vi "Disabled.vi"(7 "Robot Mode":T2, 10 "Match Info":T1={"Autonomous Elapsed Seconds"=0.0, "TeleOp Elapsed Seconds"=0.0, "Disabled Elapsed Seconds"=0.0, "Visited Autonomous"=FALSE, "Visited TeleOp"=FALSE, "Visited Disabled"=FALSE, "Autonomous Settings"={"Autonomous Style"=enum."Independent", "VI Refnum"=refnum}}, 11 "Call Context":T3) -> ()   [LabVIEW 2013]
doc: "This VI is called each time a disabled packet is received from the DS. It is often used to prepare for the next robot mode, to calibrate sensors, etc."
uses:
  <vilib>/Rock Robotics/WPI/DriverStation/WPI_DriverStationDerivedRobotMode.ctl
  <vilib>/Rock Robotics/WPI/DriverStation/WPI_DriverStationRobotMode2.ctl
  <vilib>/Rock Robotics/WPI/DriverStation/WPI_DriverStationMatch Info.ctl
  Rollers/Roller Control.ctl
  Rollers/Roller Mode.ctl
  Common Code/Change Detect Boolean.vi
  <vilib>/Rock Robotics/WPI/Joystick/WPI_JoystickRefNum Registry Get.vi
  Utilities/Invert Joystick Y Axes.vi
  Drivetrain/Drivetrain Set.vi
  Robot Global Data.vi
  <vilib>/Rock Robotics/WPI/Joystick/WPI_JoystickGet.vi
  <vilib>/Rock Robotics/WPI/Joystick/WPI_JoystickGetSetRefNum.vi
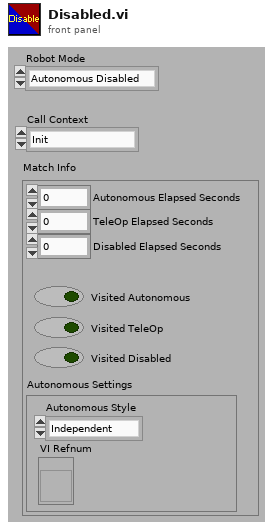
[diagram p1: front panel]
types:
  T1 = typedef "WPI_DriverStationMatch Info.ctl" = cluster{"Autonomous Elapsed Seconds":dbl, "TeleOp Elapsed Seconds":dbl, "Disabled Elapsed Seconds":dbl, "Visited Autonomous":bool, "Visited TeleOp":bool, "Visited Disabled":bool, "Autonomous Settings":cluster{"Autonomous Style":enum16{"Iterative", "Independent"}, "VI Refnum":refnum<vi>}}
  T2 = typedef "WPI_DriverStationRobotMode2.ctl" = enum16{"Autonomous Disabled", "Autonomous Enabled", "Teleop Disabled", "Teleop Enabled", "Timeout", "Finish", "Test Disabled", "Test Enabled"}
  T3 = typedef "WPI_DriverStationDerivedRobotMode.ctl" = enum16{"Init", "Execute", "Stop"}
  T4 = typedef "Roller Control.ctl" = cluster{"Mode":T5, "Front":enum16{"Stop", "Forward", "Reverse"}, "Back":enum16{"Stop", "Forward", "Reverse"}, "Reset":bool, "Front Piston":bool, "Halo":bool, "Net Piston":bool, "Carry Two":bool, "Hold":bool}
  T5 = typedef "Roller Mode.ctl" = enum16{"None", "Front", "Back", "Both", "Manual"}
  T6 = typedef "WPI_JoystickButtonState.ctl" = cluster{"Button 1":bool, "Button 2":bool, "Button 3":bool, "Button 4":bool, "Button 5":bool, "Button 6":bool, "Button 7":bool, "Button 8":bool, "Button 9":bool, "Button 10":bool, "Button 11":bool, "Button 12":bool}
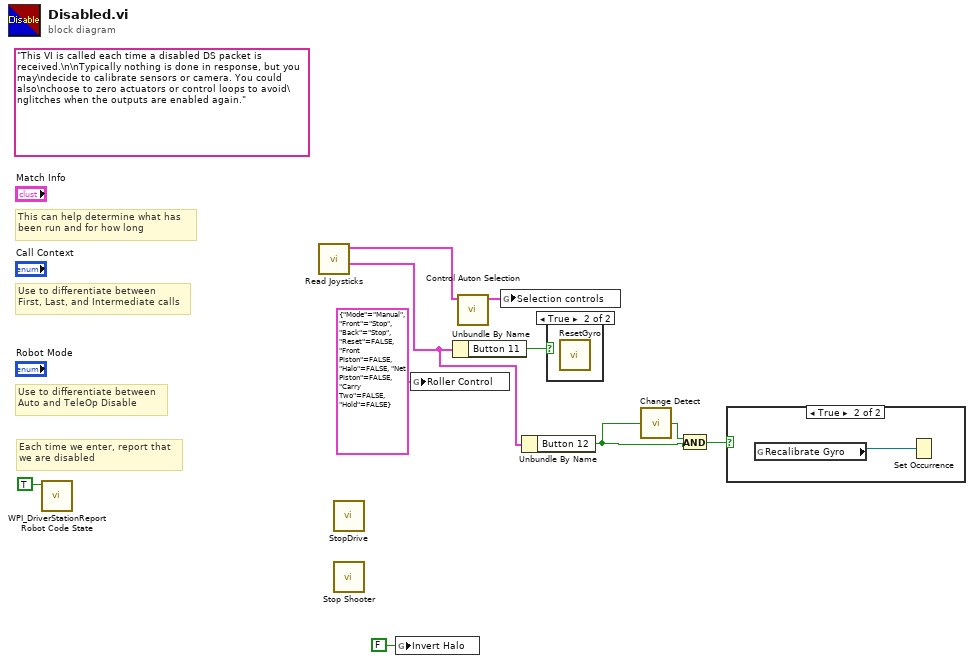
[diagram p0: block diagram]
diagram:
  (unwired) "This VI is called each time a disabled DS packet is received.\n\nTypically nothing is done in response, but you may\ndecide to calibrate sensors or camera. You could also\nchoose to zero actuators or control loops to avoid\nglitches when the outputs are enabled again."
  # "Each time we enter, report that\nwe are disabled"
  # "Use to differentiate between\nFirst, Last, and Intermediate calls"
  # "This can help determine what has\nbeen run and for how long"
  # "Use to differentiate between\nAuto and TeleOp Disable"
  n1 = call <vilib>:"WPI_DriverStationReport Robot Code State.vi"("Disabled"=TRUE ("Autonomous")) -> ()  [unwired: 10 in, 1 out]
  n2 = call "Read Joysticks.vi"() -> ("Manipulator Buttons"=w2:T6, "Driver Buttons"=w6:T6)  [unwired: 8 in, 2 out]
  n3 = call "StopDrive.vi"() -> ()  [unwired: 12 in]
  n4 = call "Stop Shooter.vi"() -> ()  [unwired: 12 in]
  n5 = global write "Robot Global Data.vi" "Invert Halo"(FALSE ("Invert Halo")) -> ()
  n6 = global write "Robot Global Data.vi" "Roller Control"(T4 {"Mode"=enum."Manual", "Front"=enum."Stop", "Back"=enum."Stop", "Reset"=FALSE, "Front Piston"=FALSE, "Halo"=FALSE, "Net Piston"=FALSE, "Carry Two"=FALSE, "Hold"=FALSE} ("Roller Command")) -> ()
  n7 = Unbundle By Name(w2) -> ("Button 11"=w9:bool)
  n8 = call "Control Auton Selection.vi"("Driver Buttons"=w6) -> ("Selection controls"=w7:cluster{"Up":bool, "Down":bool})  [unwired: 10 in]
  n9 = global write "Robot Global Data.vi" "Selection controls"(w7) -> ()
  n10 = Unbundle By Name(w2) -> ("Button 12"=w3:bool)
  n11 = case shown="True" w9 {
    frame False {
    }
    frame True {
      n12 = call "ResetGyro.vi"() -> ()  [unwired: 12 in]
    }
  }
  n13 = call-poly "Change Detect.vi"("In"=w3) -> ("Changed?"=w4:bool)
  n14 = And(x=w4, y=w3) -> (x .and. y?=w5:bool)
  n15 = case shown="True" w5 {
    frame False {
    }
    frame True {
      n16 = global read "Robot Global Data.vi" "Recalibrate Gyro"() -> (w11:refnum<k4>)
      n17 = Set Occurrence(w11) -> ()
    }
  }
